vi "GetEquipment.vi"(8 "error in (no error)":errorcluster, 10 "id":string, 11 "equipment list":T1[](array[typedef])) -> (0 "error out":errorcluster, 1 "found":bool, 2 "equipment":T1)   [LabVIEW 2017, in "DeviceModelHelpers.lvlib"]
doc: "Returns the properties of a specific equipment node in the cluster from the Get Equipment List VI."
uses:
  <vilib>/addons/InsightCM/Utilities/DeviceModelHelpers/DeviceModelHelpers.lvlib
  <vilib>/addons/InsightCM/MessageBus/Base/controls/Equipment.ctl
  <vilib>/addons/InsightCM/MessageBus/Base/controls/KeyValuePair.ctl
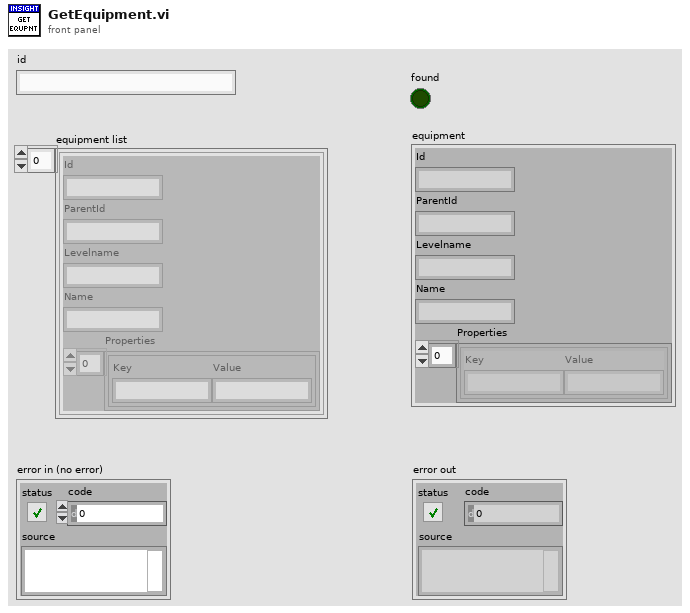
[diagram p1: front panel]
types:
  T1 = typedef "Equipment.ctl" = cluster{"Id":string, "ParentId":string, "Levelname":string, "Name":string, "Properties":T2[]}
  T2 = typedef "KeyValuePair.ctl" = cluster{"Key":string, "Value":string}
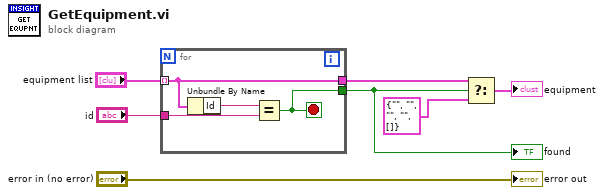
[diagram p0: block diagram]
diagram:
  n1 = for {
    tunnel: "equipment list" -> [w8] mode=indexing
    tunnel: "id" -> [w10]
    tunnel: [w9] -> w4
    tunnel: [w8] -> w3
    stop <- w9 stop-if-true
    n2 = Unbundle By Name(w8) -> ("Id"=w11:string)
    n3 = Equal?(x=w11, y=w10) -> (x = y?=w9:bool)
  }
  "found" <- w4
  n4 = Select(t=w3, s=w4, f=T1 {"Id"="", "ParentId"="", "Levelname"="", "Name"="", "Properties"=[]}) -> (s? t:f=→"equipment":T1)
  "error out" <- "error in (no error)"
